vi "test_Timestamp (Date only).vi"(8 "error in (no error)":errorcluster, 11 "TestCase in":refnum<class "Test Read File.lvclass">) -> (0 "error out":errorcluster, 3 "TestCase out":refnum<class "Test Read File.lvclass">)   [LabVIEW 2019, in "Test Read File.lvclass"]
uses:
  Test Read File.lvclass
  C:/Program Files/National Instruments/LabVIEW 2024/vi.lib/Astemes/LUnit/Test Case.lvclass
  Test Read File.lvclass/Test Read File.ctl
  <vilib>/Astemes/LUnit/Test Case.lvclass/Test Case.ctl
  893642d9-d86c-4e14-8998-c045412cc661.vi
  <vilib>/Astemes/LUnit/Core/LUnit Test Case/Private/Append Pass Result.vi
  <vilib>/Astemes/LUnit/Core/LUnit Test Case/Private/Append Fail Result.vi
  893642d9-d86c-4e14-8998-c045412cc661.vi/9c5d11cd-9439-4240-a1ee-d9baace9c924.vi
  <vilib>/Astemes/LUnit/Core/LUnit Test Case/Private/Run In UI.vi
  <vilib>/Utility/error.llb/Clear Errors.vi
  Read/Read Section - Timestamp.vi
  TSC File IO.lvlib
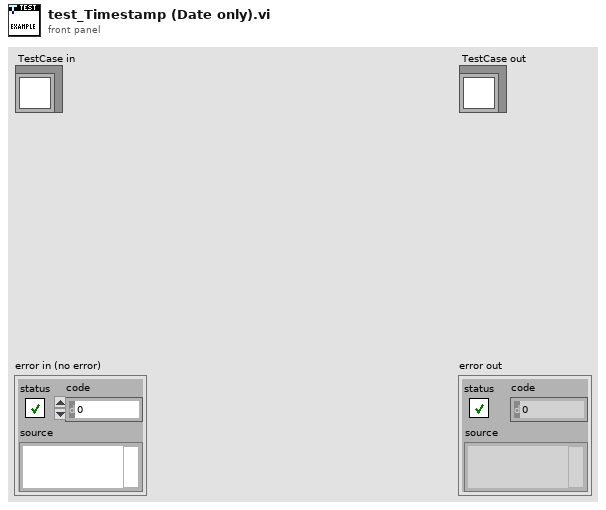
[diagram p1: front panel]
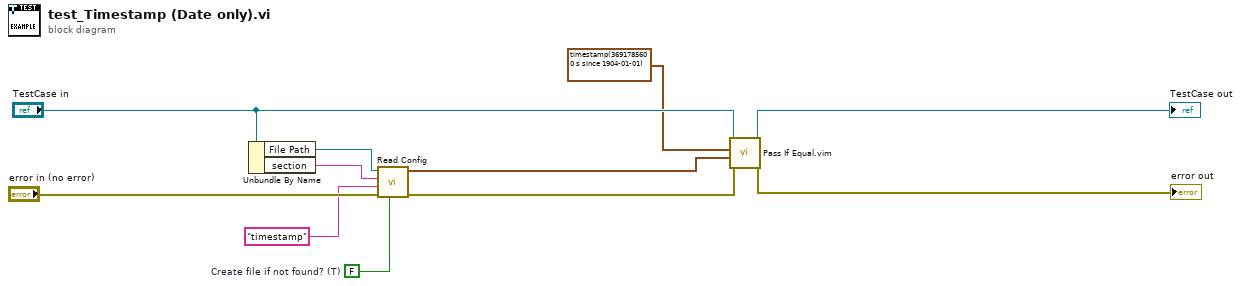
[diagram p0: block diagram]
diagram:
  w2 = FALSE  # Create file if not found? (T)
  n1 = Unbundle By Name("TestCase in") -> ("File Path"=w6:path, "section"=w5:string)
  n2 = call-poly "Read Config.vi"("Create file if not found? (T)"=w2, "error in (no error)"="error in (no error)", "key"="timestamp", "section"=w5, "Path"=w6) -> ("error out"=w7:errorcluster, "Value"=w4:timestamp)  [unwired: 5 in]
  n3 = call "Pass If Equal.vim"("error in (no error)"=w7, "Actual"=w4, "Expected"=timestamp(3691785600 s since 1904-01-01) ("Value"), "LUnit Test Case In"="TestCase in") -> ("error out"=→"error out":errorcluster, "LUnit Test Case Out"=→"TestCase out":refnum<class "Test Read File.lvclass">)  [unwired: 6 in]
